vi "Drain.vi"(0 "GEA2 Reference In":refnum<k24>, 5 "Standalone?":bool, 11 "Error In":errorcluster) -> (4 "GEA2 Reference Out":refnum<k24>, 6 "Pass/Fail?":bool, 8 "Report Text":string, 15 "Error Out":errorcluster)   [LabVIEW 2016, in "Centauro.lvlib"]
doc: "This VI performs a test to ensure the washer MC fills the tub with the appropriate amount of hot and cold water."
uses:
  Projects/Centauro.lvlib
  Q:/Common/DLLs/GEA3/GeaCommunication.dll
  Common/DLLs/GEA3/GeaCommunication.dll
  Common/LabVIEW GEA2 Toolkit/LabVIEW_GEA2_Toolkit.lvlibp/type defs/Source_Destination.ctl
  Common/LabVIEW GEA2 Toolkit/LabVIEW_GEA2_Toolkit.lvlibp/type defs/ERD Write Data In.ctl
  Common/LabVIEW GEA2 Toolkit/LabVIEW_GEA2_Toolkit.lvlibp/type defs/Data Type.ctl
  Common/LabVIEW GEA2 Toolkit/LabVIEW_GEA2_Toolkit.lvlibp/type defs/ERD Read Data In.ctl
  <vilib>/DAQmx/read.llb/DAQmx Read (Digital Bool 1Line 1Point).vi
  <vilib>/DAQmx/create/channels.llb/DAQmx Create Channel (DI-Digital Input).vi
  <vilib>/DAQmx/miscellaneous.llb/DAQmx Fill In Error Info.vi
  Common/LabVIEW GEA2 Toolkit/LabVIEW_GEA2_Toolkit.lvlibp
panel:
  in  "GEA Inputs":T1={"Source"=228, "Destination"=32} {"Destination" format="%.0x"; "Source" format="%.0x"}
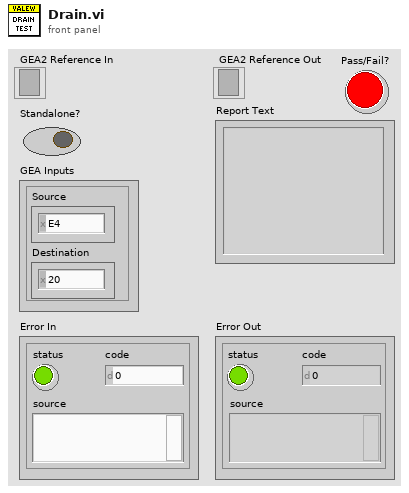
[diagram p1: front panel]
types:
  T1 = typedef "LabVIEW_GEA2_Toolkit.lvlibp/Source_Destination.ctl" = cluster{"Source":u8, "Destination":u8}
  T2 = typedef "LabVIEW_GEA2_Toolkit.lvlibp/ERD Write Data In.ctl" = cluster{"ERD Number":u16, "Data Type":T3, "Data":string}
  T3 = typedef "LabVIEW_GEA2_Toolkit.lvlibp/Data Type.ctl" = enum16{"string", "boolean", "uint8_t", "uint16_t", "uint32_t", "uint64_t", "int8_t", "int16_t", "int32_t", "int64_t"}
  T4 = typedef "LabVIEW_GEA2_Toolkit.lvlibp/ERD Read Data In.ctl" = cluster{"ERD Number":u16, "Data Type":T3}
  T5 = typedef "LabVIEW_GEA2_Toolkit.lvlibp/ERD Read Data Out.ctl" = cluster{"ERD Number":u16, "Data":string}
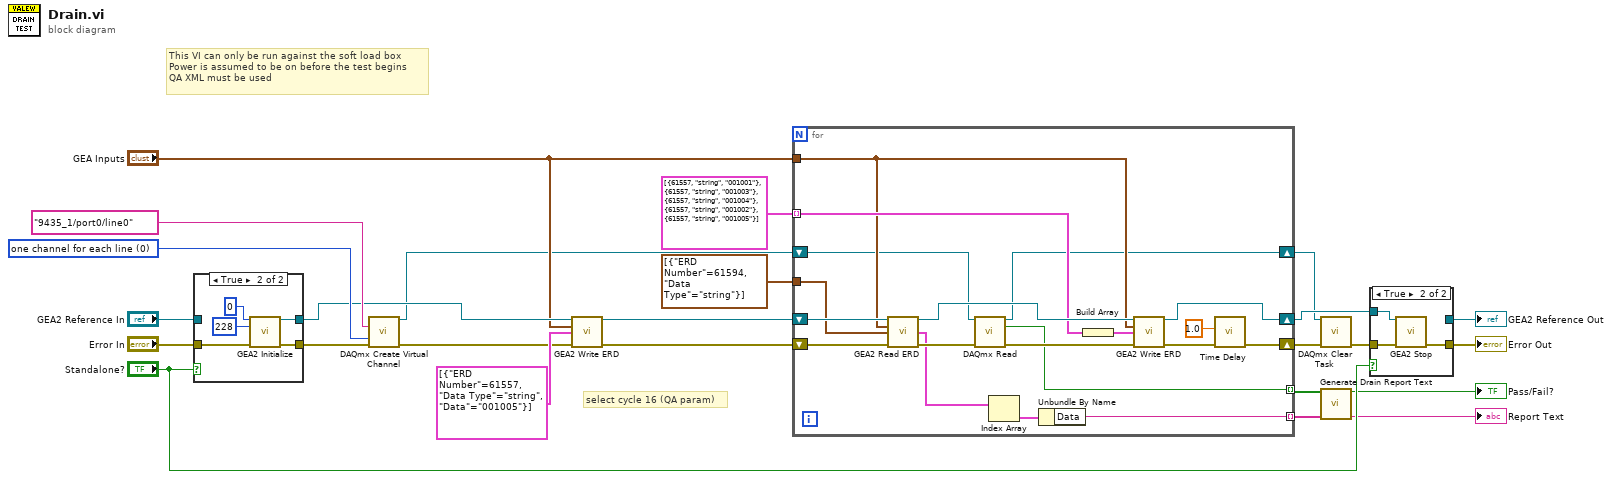
[diagram p0: block diagram]
diagram:
  w21 = 0 items=["one channel for each line", "one channel for all lines"] ("line grouping")
  # "This VI can only be run against the soft load box\nPower is assumed to be on before the test begins\nQA XML must be used"
  # "select cycle 16 (QA param)"
  n1 = case shown="True" "Standalone?" {
    tunnel: "Error In" -> [w27 w30]
    tunnel: [w26 w29] -> w17
    tunnel: [w27 w28] -> w18
    tunnel: "GEA2 Reference In" -> [w26 _]
    frame False {
    }
    frame True {
      n2 = call "GEA2 Initialize.vi"("Board Index"=0, "Source Address"=u8 228, "error in"=w30) -> ("GEA2 Reference Out"=w29:refnum<k24>, "error out"=w28:errorcluster)  [unwired: 10 in, 1 out]
    }
  }
  n3 = call-poly <vilib>:"DAQmx Create Virtual Channel.vi"("lines"=tag "9435_1/port0/line0" ("Drain Pump Line"), "line grouping"=w21, "error in"=w18) -> ("task out"=w9:refnum<k21>, "error out"=w15:errorcluster)  [unwired: 11 in]
  n4 = call "GEA2 Write ERD.vi"("GEA2 Reference In"=w17, "GEA Inputs"="GEA Inputs", "Write ERD List"=T2[] [{"ERD Number"=61557, "Data Type"=enum."string", "Data"="001005"}], "Error In"=w15) -> ("GEA2 Reference Out"=w10:refnum<k24>, "Error Out"=w11:errorcluster)  [unwired: 9 in, 1 out]
  n5 = for {
    shift-right: [w48] -> w5
    shift-left: w11 -> [w46]
    shift-right: [w47] -> w7
    shift-left: w10 -> [w45]
    tunnel: [w42] -> w4 mode=indexing
    tunnel: T2[] [{"ERD Number"=61557, "Data Type"=enum."string", "Data"="001001"}, {"ERD Number"=61557, "Data Type"=enum."string", "Data"="001003"}, {"ERD Number"=61557, "Data Type"=enum."string", "Data"="001004"}, {"ERD Number"=61557, "Data Type"=enum."string", "Data"="001002"}, {"ERD Number"=61557, "Data Type"=enum."string", "Data"="001005"}] ("Write ERD List") -> [w41] mode=indexing
    tunnel: "GEA Inputs" -> [w39]
    tunnel: T4[] [{"ERD Number"=61594, "Data Type"=enum."string"}] ("Read ERD List") -> [w33]
    shift-right: [w37] -> w6
    shift-left: w9 -> [w38]
    tunnel: [w34] -> w3 mode=indexing
    n6 = call "GEA2 Read ERD.vi"("GEA2 Reference In"=w45, "GEA Inputs"=w39, "Read ERD List"=w33, "Error In"=w46) -> ("GEA2 Reference Out"=w51:refnum<k24>, "ERD Data Out"=w36:T5[], "Error Out"=w44:errorcluster)  [unwired: 8 in, 1 out]
    n7 = call-poly <vilib>:"DAQmx Read.vi"("task/channels in"=w38, "error in"=w44) -> ("task out"=w37:refnum<k21>, "data"=w42:bool, "error out"=w43:errorcluster)  [unwired: 11 in]
    n8 = Index Array(array=w36) -> (element=w35:T5)  [unwired: 1 in]
    n9 = Unbundle By Name(w35) -> ("Data"=w34:string)
    n10 = Build Array(w41) -> (w40:T2[])
    n11 = call "GEA2 Write ERD.vi"("GEA2 Reference In"=w51, "GEA Inputs"=w39, "Write ERD List"=w40, "Error In"=w43) -> ("GEA2 Reference Out"=w47:refnum<k24>, "Error Out"=w50:errorcluster)  [unwired: 9 in, 1 out]
    n12 = call "Time Delay"("error in (no error)"=w50, "Delay Time (s)"=1.0) -> ("error out"=w48:errorcluster)  [unwired: 9 in]
  }
  n13 = call <vilib>:"DAQmx Clear Task.vi"("task in"=w6, "error in"=w5) -> ("error out"=w19:errorcluster)  [unwired: 13 in]
  n14 = call "Generate Drain Report Text.vi"("Drain State DAQ In"=w4, "Drain State ERD In"=w3) -> ("Pass/Fail?"=→"Pass/Fail?":bool, "Report Text"=→"Report Text":string)  [unwired: 12 in]
  n15 = case shown="True" "Standalone?" {
    tunnel: [w53 w56] -> w24
    tunnel: w19 -> [w53 w55]
    tunnel: [w52 _] -> w8
    tunnel: w7 -> [w52 w54]
    frame False {
    }
    frame True {
      n16 = call "GEA2 Stop.vi"("GEA2 Reference In"=w54, "Error In"=w55) -> ("Error Out"=w56:errorcluster)  [unwired: 13 in]
    }
  }
  "Error Out" <- w24
  "GEA2 Reference Out" <- w8
